vi "Launch Plot.vi"(8 "error in (no error)":errorcluster, 9 "Plot type":T1, 10 "File Path Control":path, 11 "Monitor-Pulse in":refnum<class "Monitor-Pulse.lvclass">) -> (0 "error out":errorcluster, 2 "Nested Actor's Enqueuer":refnum<class "Message Enqueuer.lvclass">, 3 "Monitor-Pulse out":refnum<class "Monitor-Pulse.lvclass">)   [LabVIEW 2016]
uses:
  Monitor-Pulse.lvclass
  C:/github/Measure_core/Controllers/Application Controller/Application Controller.lvclass
  C:/github/Measure_core/Da Base/Da Base.lvclass
  C:/Program Files/National Instruments/LabVIEW 2016/vi.lib/ActorFramework/Actor/Actor.lvclass
  Measure_core/Plots/Plot types.ctl
  <vilib>/ActorFramework/Message Enqueuer/Message Enqueuer.lvclass
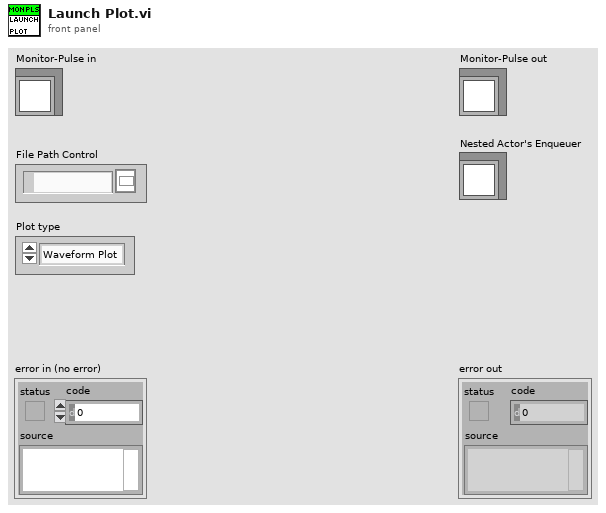
[diagram p1: front panel]
types:
  T1 = typedef "Plot types.ctl" = enum16{"Waveform Plot", "XY Plot", "Full XY"}
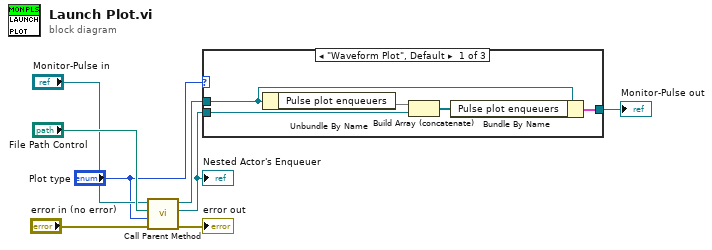
[diagram p0: block diagram]
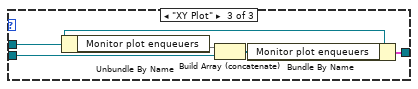
[diagram p3: hidden frame]
diagram:
  n1 = call-parent "Call Parent Method"("error in (no error)"="error in (no error)", "Plot type"="Plot type", "File Path Control"="File Path Control", "Application Controller in"="Monitor-Pulse in") -> ("error out"=→"error out":errorcluster, "Nested Actor's Enqueuer"=w2:refnum<class "Message Enqueuer.lvclass">, "Application Controller out"=w3:refnum<class "Monitor-Pulse.lvclass">)  [unwired: 5 in]
  "Nested Actor's Enqueuer" <- w2
  n2 = case shown="\"Waveform Plot\", Default" "Plot type" {
    tunnel: w3 -> [w11 w14 w17]
    tunnel: w2 -> [w12 _ w18]
    tunnel: [w9 w14 w15] -> w1
    frame "Waveform Plot", Default {
      n3 = Unbundle By Name(w11) -> ("Pulse plot enqueuers"=w13)
      n4 = Build Array (concatenate)(w13, w12) -> (w10:refnum<class "Message Enqueuer.lvclass">[])
      n5 = Bundle By Name(cluster=w11, "Pulse plot enqueuers"=w10) -> (w9:cluster{})
    }
    frame "Full XY" {
    }
    frame "XY Plot" {
      n6 = Unbundle By Name(w17) -> ("Monitor plot enqueuers"=w19)
      n7 = Build Array (concatenate)(w19, w18) -> (w16:refnum<class "Message Enqueuer.lvclass">[])
      n8 = Bundle By Name(cluster=w17, "Monitor plot enqueuers"=w16) -> (w15:cluster{})
    }
  }
  "Monitor-Pulse out" <- w1
